vi "函数类型1测试.vi"() -> ()   [LabVIEW 2010]
uses:
  全局量/试验配置信息.vi
  全局量/全局_配置.vi
panel:
  in  "配置文件列表":u16(ring)
  in  "同步_1":i32
  in  "数组_反馈值":dbl[][](array[numeric])
  in  "第几个数据":i32
  in  "第几组数据":i32
  out "数组_AD幅值":sgl[](array[numeric])
  out "数组_DSP幅值":sgl[](array[numeric])
  in  "数组_设定值":dbl[][](array[numeric])
  in  "数组_选择":bool[](array[boolean])
  out "light_32":bool
  out "light_31":bool
  out "light_30":bool
  out "light_29":bool
  out "light_28":bool
  out "light_27":bool
  out "light_26":bool
  out "light_25":bool
  out "light_24":bool
  out "light_23":bool
  out "light_22":bool
  out "light_21":bool
  out "light_20":bool
  out "light_19":bool
  out "light_18":bool
  out "light_17":bool
  out "Analog_back":string[][](table) caption="表格"
  in  "A_32":bool
  in  "A_31":bool
  in  "A_30":bool
  in  "A_29":bool
  in  "A_28":bool
  in  "A_27":bool
  in  "A_26":bool
  in  "A_25":bool
  in  "A_24":bool
  in  "A_23":bool
  in  "A_22":bool
  in  "A_21":bool
  in  "A_20":bool
  in  "A_19":bool
  in  "A_18":bool
  in  "A_17":bool
  out "合格？":bool[][](array[boolean])
  out "测试结论":string
  out "light_16":bool
  out "light_15":bool
  out "light_14":bool
  out "light_13":bool
  out "light_12":bool
  out "light_11":bool
  out "light_10":bool
  out "light_9":bool
  out "light_8":bool
  out "light_7":bool
  out "light_6":bool
  out "light_5":bool
  out "light_4":bool
  out "light_3":bool
  out "light_2":bool
  out "light_1":bool
  out "退出？":bool
  in  "btn_反选":bool
  in  "btn_全选":bool
  in  "A_16":bool
  in  "A_15":bool
  in  "A_14":bool
  in  "A_13":bool
  in  "A_12":bool
  in  "A_11":bool
  in  "A_10":bool
  in  "A_9":bool
  in  "A_8":bool
  in  "A_7":bool
  in  "A_6":bool
  in  "A_5":bool
  in  "A_4":bool
  in  "A_3":bool
  in  "A_2":bool
  in  "A_1":bool
  in  "btn_取消":bool
  in  "btn_开始测试":bool
  in  "Analog_IN":string[][](table) caption="表格"
  out "Analog_WC":string[][](table) caption="表格"
  # "模拟量选择及输入值（V）"
  # "模拟量反馈值（V）"
  # "模拟量误差值（%）"
  # "加载配置文件："
  # "测试结论："
  # "从0开始"
  # "从1开始,第0列没有使用"
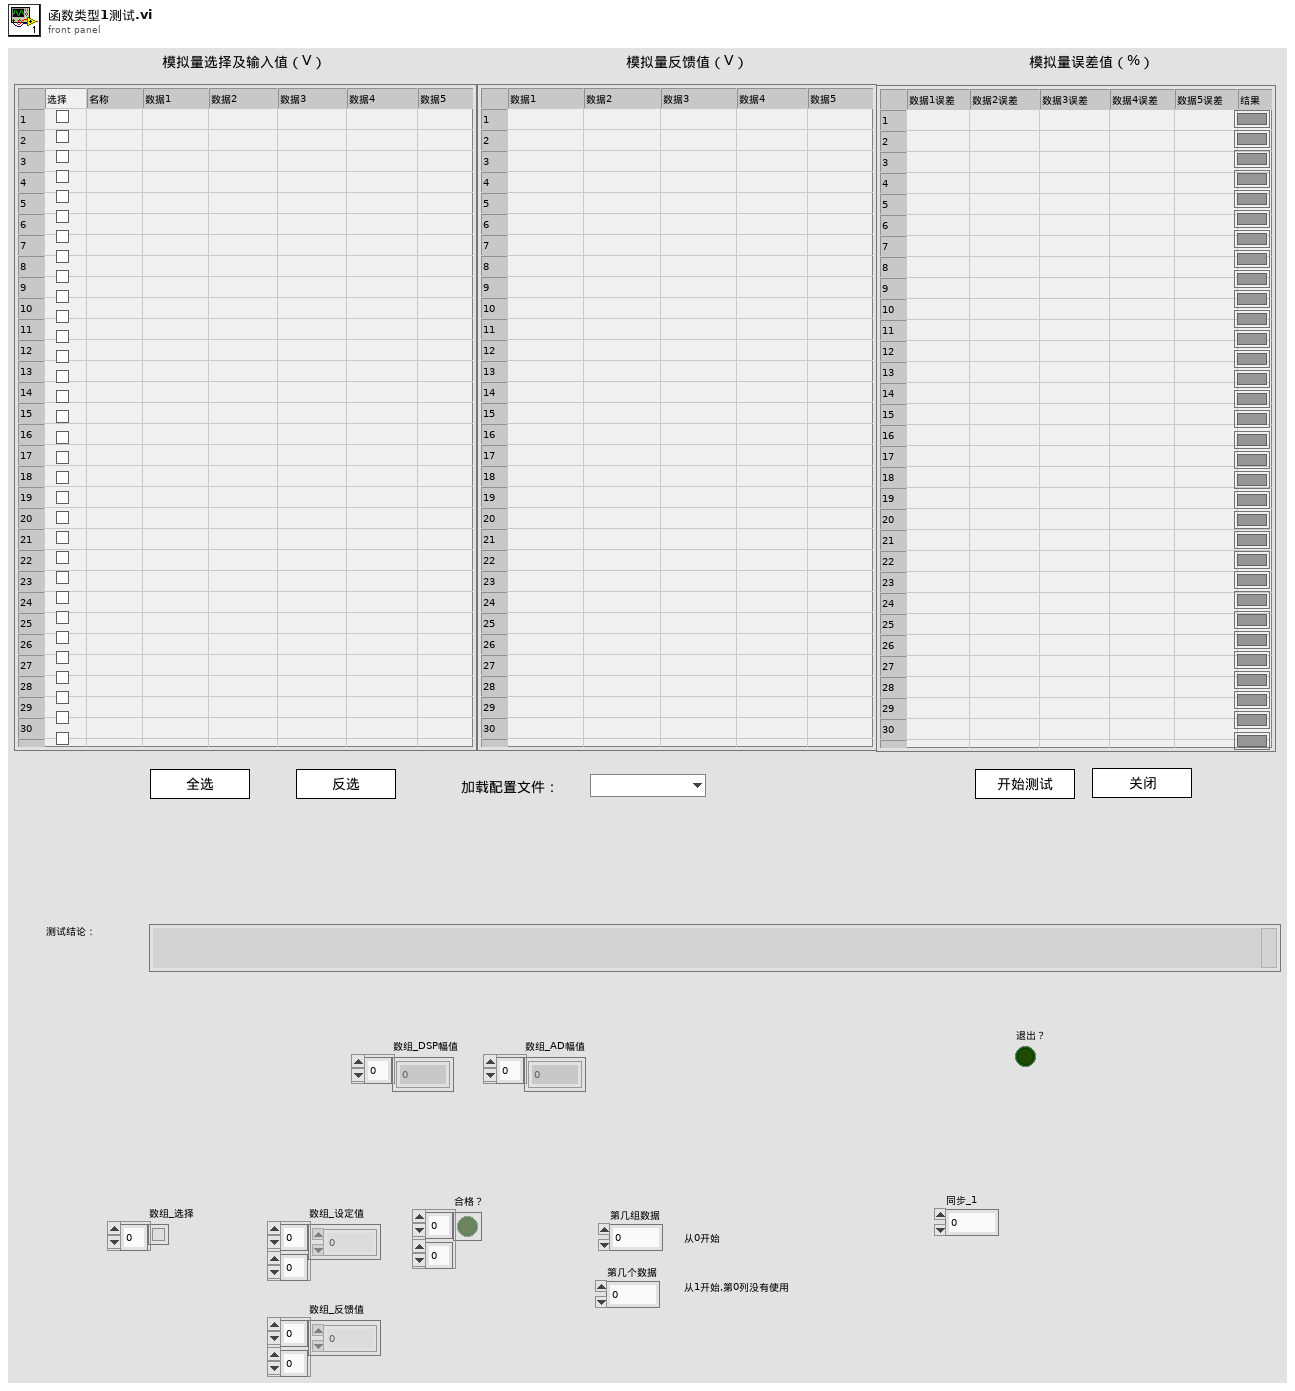
[diagram p1: front panel]
types:
  T1 = enum8{"Enabled", "Disabled", "Disabled and Grayed Out"}
  T2 = cluster{"数字量输入信号路数":u32, "数字量输出信号路数":u32, "DSP模拟量输入信号路数":u32, "DSP模拟量输入信号幅值":u32, "AD模拟量输入信号路数":u32, "AD模拟量输入信号幅值":u32, "RS232端口":u32, "RS232通信路数":u32, "RS232波特率":u32, "RS485端口":u32, "RS485通信路数":u32, "RS485波特率":u32, "CAN通信端口":string, "CAN波特率":u32, "以太网选择?":bool, "控制板IP":string, "以太网端口":u32}
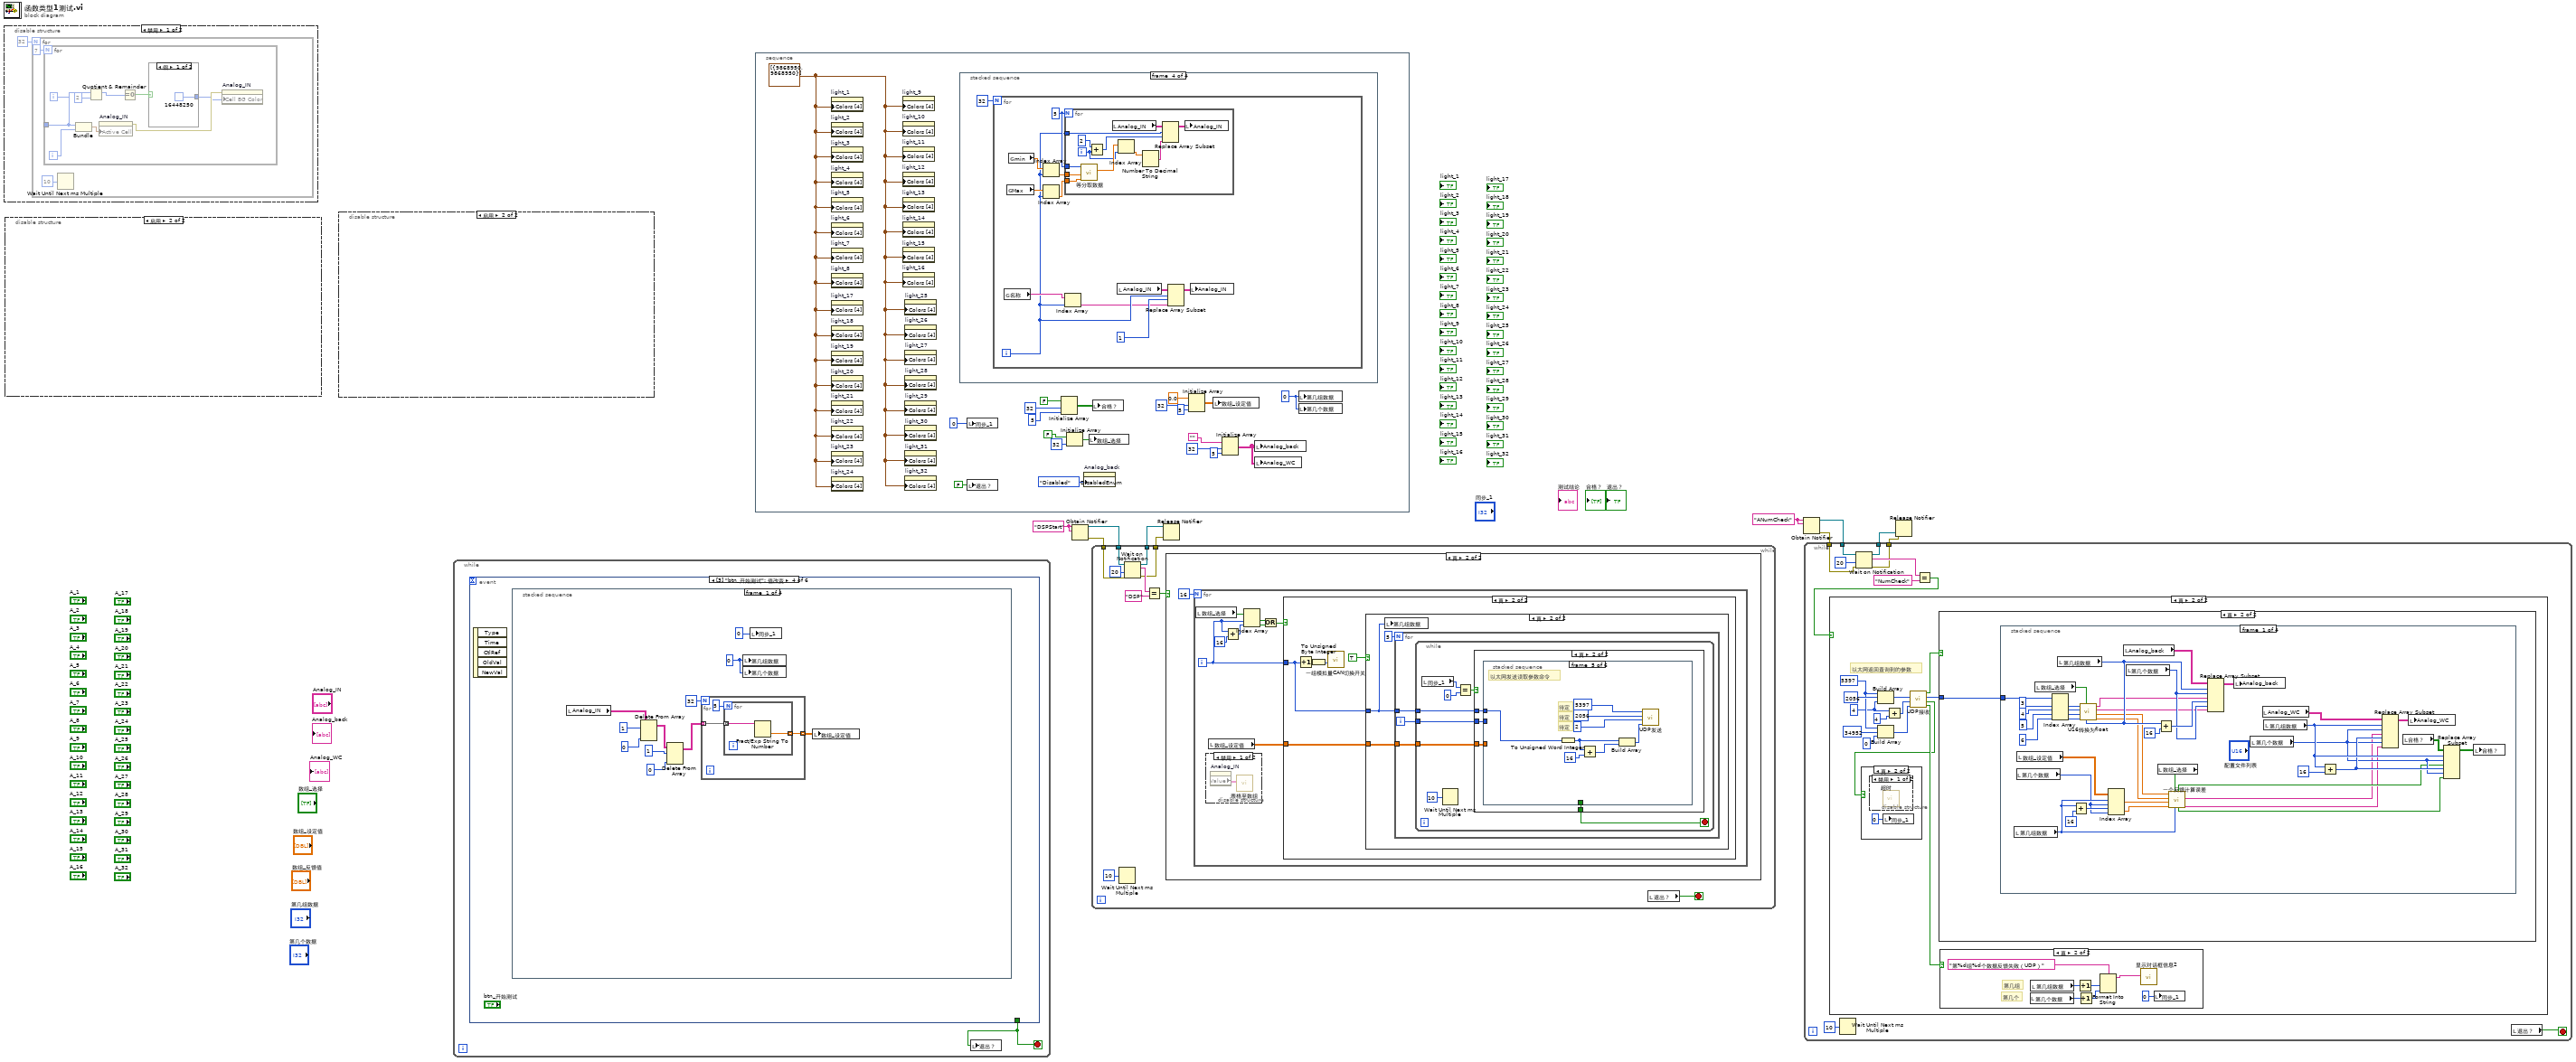
[diagram p0: block diagram]
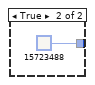
[diagram p2: hidden frame]
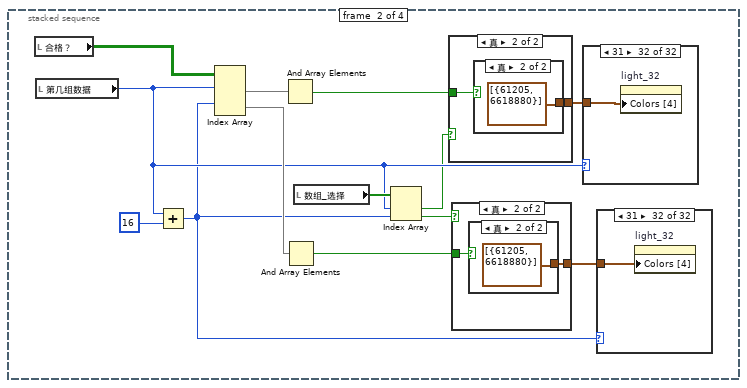
[diagram p9: hidden frame]
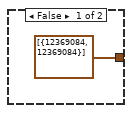
[diagram p10: hidden frame]
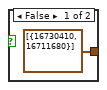
[diagram p11: hidden frame]
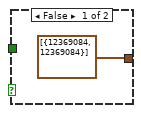
[diagram p12: hidden frame]
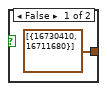
[diagram p13: hidden frame]
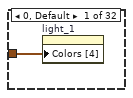
[diagram p14: hidden frame]
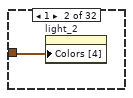
[diagram p15: hidden frame]
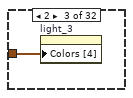
[diagram p16: hidden frame]
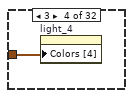
[diagram p17: hidden frame]
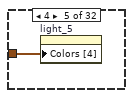
[diagram p18: hidden frame]
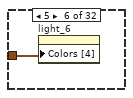
[diagram p19: hidden frame]
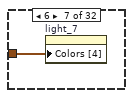
[diagram p20: hidden frame]
diagram:
  w5 = "ANumCheck" ("名称（未命名）")
  w8 = "DSPStart" ("名称（未命名）")
  n1 = disable-structure shown="禁用" {
    frame Disabled {
      n2 = for {
        N: 32 -> [_]
        i -> [w13]
        n3 = for {
          N: 7 -> [_]
          tunnel: w13 -> [w21]
          i -> [w15]
          n4 = Bundle(w21, w15) -> (w18:cluster{i32, i32})  [unwired: 1 in]
          n5 = Quotient & Remainder(x=w21, y=2) -> (x-y*floor(x/y)=w19:i32)  [unwired: 1 out]
          n6 = property on="Analog_IN" class="Tbl (严格)"("Active Cell"=w18) -> (error out=w17:errorcluster)  [unwired: 2 in, 1 out]
          n7 = Equal To 0?(x=w19) -> (x = 0?=w22:bool)
          n8 = case shown="假" w22 {
            tunnel: [u32 16448250 u32 15723488] -> w16
            frame False {
            }
            frame True {
            }
          }
          n9 = property on="Analog_IN" class="Tbl (严格)"(error in=w17, "Cell BG Color"=w16) -> ()  [unwired: 1 in, 2 out]
        }
        n10 = Wait Until Next ms Multiple(millisecond multiple=u32 10 ("毫秒倍数")) -> ()  [unwired: 1 out]
      }
    }
    frame Enabled {
    }
  }
  n11 = disable-structure shown="启用" {
    frame Disabled {
      n12 = for {
        N: 32 -> [_]
        i -> [w26]
        n13 = for {
          N: 7 -> [_]
          tunnel: w26 -> [w29]
          i -> [w30]
          n14 = Bundle(w29, w30) -> (w33:cluster{i32, i32})  [unwired: 1 in]
          n15 = property on="Analog_IN" class="Tbl (严格)"("Active Cell"=w33) -> (error out=w31:errorcluster)  [unwired: 2 in, 1 out]
          n16 = property on="Analog_IN" class="Tbl (严格)"(error in=w31, "Justify"=enum16{"Left", "Center", "Right"}."Left" ("活动单元格:单元格对齐")) -> ()  [unwired: 1 in, 2 out]
        }
        n17 = Wait Until Next ms Multiple(millisecond multiple=u32 10 ("毫秒倍数")) -> ()  [unwired: 1 out]
      }
    }
    frame Enabled {
    }
  }
  n18 = disable-structure shown="启用" {
    frame Disabled {
      n19 = for {
        N: 32 -> [_]
        i -> [w39]
        n20 = Wait Until Next ms Multiple(millisecond multiple=u32 10 ("毫秒倍数")) -> ()  [unwired: 1 out]
        n21 = Bundle(w39, 1) -> (w38:cluster{i32, i32})  [unwired: 1 in]
        n22 = property on="Analog_IN" class="Tbl (严格)"("Active Cell"=w38) -> (error out=w35:errorcluster)  [unwired: 2 in, 1 out]
        n23 = property on="Analog_IN" class="Tbl (严格)"(error in=w35, "DisabledEnum"=T1."Enabled" ("禁用")) -> ()  [unwired: 1 in, 2 out]
      }
    }
    frame Enabled {
    }
  }
  n24 = while {
    stop <- w41 stop-if-true
    n25 = event shown="[3] \"btn_开始测试\": 值改变" {
      selector: _ -> [_ _ _ _ _ _]
      dyn-events: _ -> [_ _ _ _ _ _]
      timeout: _ -> [_ _ _ _ _ _]
      tunnel: [_ TRUE TRUE _ _ _] -> w41
      event Timeout {
        n26 = event-data() -> ()  [unwired: 1 in, 2 out]
      }
      event Panel Close {
        n27 = event-data() -> ()  [unwired: 1 in, 3 out]
      }
      event "btn_取消": Value Change {
        n28 = event-data() -> ()  [unwired: 1 in, 5 out]
      }
      event "btn_开始测试": Value Change {
        n29 = event-data() -> ()  [unwired: 1 in, 5 out]
        n30 = stacked-sequence {
          frame #0 {
            w48 = 0 ("第几组数据")
            n31 = local read "Analog_IN"() -> (w54:string[][])
            n32 = Delete From Array(array=w54, length=1 ("长度"), index (col)=0 ("禁用的索引 (列)")) -> (array with subset deleted=w46:string[][])  [unwired: 1 in, 1 out]
            n33 = Delete From Array(array=w46, length=1 ("长度"), index (col)=0 ("禁用的索引 (列)")) -> (array with subset deleted=w44:string[][])  [unwired: 1 in, 1 out]
            n34 = for {
              N: 32 -> [_]
              tunnel: w44 -> [w57] mode=indexing
              tunnel: [w56] -> w53 mode=indexing
              n35 = for {
                N: 5 -> [_]
                tunnel: w57 -> [w59] mode=indexing
                tunnel: [w58] -> w56 mode=indexing
                n36 = Fract/Exp String To Number(string=w59) -> (number=w58:dbl)  [unwired: 3 in, 1 out]
              }
            }
            n37 = local write "第几组数据"(w48) -> ()
            n38 = local write "第几个数据"(w48) -> ()
            n39 = local write "同步_1"(0 ("同步_2")) -> ()
            n40 = local write "数组_设定值"(w53) -> ()
          }
          frame #1 {
            n41 = local read "Analog_back"() -> (w62:string[][])
            n42 = local read "Analog_WC"() -> (w61:string[][])
            n43 = for {
              tunnel: w61 -> [w98] mode=indexing
              i -> [w97]
              n44 = for {
                tunnel: w98 -> [_] mode=indexing
                tunnel: w97 -> [w102]
                i -> [w101]
                n45 = local read "Analog_WC"() -> (w103:string[][])
                n46 = Replace Array Subset(array=w103, new element="", index (row)=w102, index (col)=w101) -> (w99:string[][])
                n47 = local write "Analog_WC"(w99) -> ()
              }
            }
            n48 = for {
              tunnel: w62 -> [w105] mode=indexing
              i -> [w104]
              n49 = for {
                tunnel: w105 -> [_] mode=indexing
                tunnel: w104 -> [w109]
                i -> [w108]
                n50 = local read "Analog_back"() -> (w110:string[][])
                n51 = Replace Array Subset(array=w110, new element="", index (row)=w109, index (col)=w108) -> (w106:string[][])
                n52 = local write "Analog_back"(w106) -> ()
              }
            }
            n53 = for {
              N: 32 -> [_]
              i -> [w64]
              n54 = case shown="31" w64 {
                tunnel: cluster{u32, u32}[] [{9868950, 9868950}] -> [w65 w66 w67 w68 w69 w70 w71 w72 w73 w74 w75 w76 w77 w78 w79 w80 w81 w82 w83 w84 w85 w86 w87 w88 w89 w90 w91 w92 w93 w94 w95 w96]
                frame 0, Default {
                  n55 = property on="light_1" class="Bool (严格)"("Colors [4]"=w65) -> ()  [unwired: 2 in, 2 out]
                }
                frame 1 {
                  n56 = property on="light_2" class="Bool (严格)"("Colors [4]"=w66) -> ()  [unwired: 2 in, 2 out]
                }
                frame 2 {
                  n57 = property on="light_3" class="Bool (严格)"("Colors [4]"=w67) -> ()  [unwired: 2 in, 2 out]
                }
                frame 3 {
                  n58 = property on="light_4" class="Bool (严格)"("Colors [4]"=w68) -> ()  [unwired: 2 in, 2 out]
                }
                frame 4 {
                  n59 = property on="light_5" class="Bool (严格)"("Colors [4]"=w69) -> ()  [unwired: 2 in, 2 out]
                }
                frame 5 {
                  n60 = property on="light_6" class="Bool (严格)"("Colors [4]"=w70) -> ()  [unwired: 2 in, 2 out]
                }
                frame 6 {
                  n61 = property on="light_7" class="Bool (严格)"("Colors [4]"=w71) -> ()  [unwired: 2 in, 2 out]
                }
                frame 7 {
                  n62 = property on="light_8" class="Bool (严格)"("Colors [4]"=w72) -> ()  [unwired: 2 in, 2 out]
                }
                frame 8 {
                  n63 = property on="light_9" class="Bool (严格)"("Colors [4]"=w73) -> ()  [unwired: 2 in, 2 out]
                }
                frame 9 {
                  n64 = property on="light_10" class="Bool (严格)"("Colors [4]"=w74) -> ()  [unwired: 2 in, 2 out]
                }
                frame 10 {
                  n65 = property on="light_11" class="Bool (严格)"("Colors [4]"=w75) -> ()  [unwired: 2 in, 2 out]
                }
                frame 11 {
                  n66 = property on="light_12" class="Bool (严格)"("Colors [4]"=w76) -> ()  [unwired: 2 in, 2 out]
                }
                frame 12 {
                  n67 = property on="light_13" class="Bool (严格)"("Colors [4]"=w77) -> ()  [unwired: 2 in, 2 out]
                }
                frame 13 {
                  n68 = property on="light_14" class="Bool (严格)"("Colors [4]"=w78) -> ()  [unwired: 2 in, 2 out]
                }
                frame 14 {
                  n69 = property on="light_15" class="Bool (严格)"("Colors [4]"=w79) -> ()  [unwired: 2 in, 2 out]
                }
                frame 15 {
                  n70 = property on="light_16" class="Bool (严格)"("Colors [4]"=w80) -> ()  [unwired: 2 in, 2 out]
                }
                frame 16 {
                  n71 = property on="light_17" class="Bool (严格)"("Colors [4]"=w81) -> ()  [unwired: 2 in, 2 out]
                }
                frame 17 {
                  n72 = property on="light_18" class="Bool (严格)"("Colors [4]"=w82) -> ()  [unwired: 2 in, 2 out]
                }
                frame 18 {
                  n73 = property on="light_19" class="Bool (严格)"("Colors [4]"=w83) -> ()  [unwired: 2 in, 2 out]
                }
                frame 19 {
                  n74 = property on="light_20" class="Bool (严格)"("Colors [4]"=w84) -> ()  [unwired: 2 in, 2 out]
                }
                frame 20 {
                  n75 = property on="light_21" class="Bool (严格)"("Colors [4]"=w85) -> ()  [unwired: 2 in, 2 out]
                }
                frame 21 {
                  n76 = property on="light_22" class="Bool (严格)"("Colors [4]"=w86) -> ()  [unwired: 2 in, 2 out]
                }
                frame 22 {
                  n77 = property on="light_23" class="Bool (严格)"("Colors [4]"=w87) -> ()  [unwired: 2 in, 2 out]
                }
                frame 23 {
                  n78 = property on="light_24" class="Bool (严格)"("Colors [4]"=w88) -> ()  [unwired: 2 in, 2 out]
                }
                frame 24 {
                  n79 = property on="light_25" class="Bool (严格)"("Colors [4]"=w89) -> ()  [unwired: 2 in, 2 out]
                }
                frame 25 {
                  n80 = property on="light_26" class="Bool (严格)"("Colors [4]"=w90) -> ()  [unwired: 2 in, 2 out]
                }
                frame 26 {
                  n81 = property on="light_27" class="Bool (严格)"("Colors [4]"=w91) -> ()  [unwired: 2 in, 2 out]
                }
                frame 27 {
                  n82 = property on="light_28" class="Bool (严格)"("Colors [4]"=w92) -> ()  [unwired: 2 in, 2 out]
                }
                frame 28 {
                  n83 = property on="light_29" class="Bool (严格)"("Colors [4]"=w93) -> ()  [unwired: 2 in, 2 out]
                }
                frame 29 {
                  n84 = property on="light_30" class="Bool (严格)"("Colors [4]"=w94) -> ()  [unwired: 2 in, 2 out]
                }
                frame 30 {
                  n85 = property on="light_31" class="Bool (严格)"("Colors [4]"=w95) -> ()  [unwired: 2 in, 2 out]
                }
                frame 31 {
                  n86 = property on="light_32" class="Bool (严格)"("Colors [4]"=w96) -> ()  [unwired: 2 in, 2 out]
                }
              }
            }
          }
          frame #2 {
            n87 = for {
              N: 32 -> [_]
              i -> [w113]
              n88 = disable-structure shown="禁用" {
                frame Disabled {
                  n89 = Wait Until Next ms Multiple(millisecond multiple=u32 10 ("毫秒倍数")) -> ()  [unwired: 1 out]
                }
                frame Enabled {
                }
              }
              n90 = for {
                N: 6 -> [_]
                tunnel: w113 -> [w121]
                i -> [w118]
                n91 = Bundle(w121, w118) -> (w117:cluster{i32, i32})  [unwired: 1 in]
                n92 = Quotient & Remainder(x=w121, y=2) -> (x-y*floor(x/y)=w119:i32)  [unwired: 1 out]
                n93 = property on="Analog_WC" class="Tbl (严格)"("Active Cell"=w117) -> (error out=w116:errorcluster)  [unwired: 2 in, 1 out]
                n94 = Equal To 0?(x=w119) -> (x = 0?=w122:bool)
                n95 = case shown="假" w122 {
                  tunnel: [u32 16448250 u32 15723488] -> w115
                  frame False {
                  }
                  frame True {
                  }
                }
                n96 = property on="Analog_WC" class="Tbl (严格)"(error in=w116, "Cell BG Color"=w115) -> ()  [unwired: 1 in, 2 out]
              }
            }
          }
          frame #3 {
            n97 = local read "A_10"() -> (w153:bool)
            n98 = local read "A_11"() -> (w152:bool)
            n99 = local read "A_12"() -> (w151:bool)
            n100 = local read "A_13"() -> (w150:bool)
            n101 = local read "A_14"() -> (w149:bool)
            n102 = local read "A_15"() -> (w148:bool)
            n103 = local read "A_16"() -> (w147:bool)
            n104 = local read "A_17"() -> (w146:bool)
            n105 = local read "A_18"() -> (w145:bool)
            n106 = local read "A_19"() -> (w144:bool)
            n107 = local read "A_20"() -> (w143:bool)
            n108 = local read "A_21"() -> (w142:bool)
            n109 = local read "A_22"() -> (w141:bool)
            n110 = local read "A_23"() -> (w140:bool)
            n111 = local read "A_24"() -> (w139:bool)
            n112 = local read "A_25"() -> (w138:bool)
            n113 = local read "A_26"() -> (w137:bool)
            n114 = local read "A_27"() -> (w136:bool)
            n115 = local read "A_28"() -> (w135:bool)
            n116 = local read "A_29"() -> (w134:bool)
            n117 = local read "A_30"() -> (w133:bool)
            n118 = local read "A_31"() -> (w132:bool)
            n119 = local read "A_32"() -> (w131:bool)
            n120 = local read "A_1"() -> (w162:bool)
            n121 = local read "A_2"() -> (w161:bool)
            n122 = local read "A_3"() -> (w160:bool)
            n123 = local read "A_4"() -> (w159:bool)
            n124 = local read "A_5"() -> (w158:bool)
            n125 = local read "A_6"() -> (w157:bool)
            n126 = local read "A_7"() -> (w156:bool)
            n127 = local read "A_8"() -> (w155:bool)
            n128 = local read "A_9"() -> (w154:bool)
            n129 = Build Array(w162, w161, w160, w159, w158, w157, w156, w155, w154, w153, w152, w151, w150, w149, w148, w147, w146, w145, w144, w143, w142, w141, w140, w139, w138, w137, w136, w135, w134, w133, w132, w131) -> (w125:bool[])
            n130 = Or Array Elements(Boolean array=w125) -> (logical OR=w130:bool)
            n131 = case shown="真" w130 {
              frame False {
                n132 = call "显示对话框信息"() -> ()  [unwired: 10 in, 2 out]
              }
              frame True {
                w164 = "DSPStart" ("名称（未命名）")
                n133 = Obtain Notifier(name (unnamed)=w164, notification data type=w164) -> (notifier out=w163:refnum<notifier>)  [unwired: 2 in, 2 out]
                n134 = Send Notification(notification="DSP" ("通知"), notifier=w163) -> ()  [unwired: 1 in, 2 out]
              }
            }
            n135 = local write "数组_选择"(w125) -> ()
            n136 = Initialize Array(FALSE, 32 ("维数大小"), 5 ("维数大小")) -> (w126:bool[][])
            n137 = local write "合格？"(w126) -> ()
          }
        }
      }
      event "btn_全选": Value Change {
        w166 = TRUE ("单选_AD_1")
        n138 = event-data() -> ()  [unwired: 1 in, 5 out]
        n139 = local write "A_1"(w166) -> ()
        n140 = local write "A_2"(w166) -> ()
        n141 = local write "A_3"(w166) -> ()
        n142 = local write "A_4"(w166) -> ()
        n143 = local write "A_5"(w166) -> ()
        n144 = local write "A_6"(w166) -> ()
        n145 = local write "A_7"(w166) -> ()
        n146 = local write "A_8"(w166) -> ()
        n147 = local write "A_9"(w166) -> ()
        n148 = local write "A_10"(w166) -> ()
        n149 = local write "A_11"(w166) -> ()
        n150 = local write "A_12"(w166) -> ()
        n151 = local write "A_13"(w166) -> ()
        n152 = local write "A_14"(w166) -> ()
        n153 = local write "A_15"(w166) -> ()
        n154 = local write "A_16"(w166) -> ()
        n155 = local write "A_17"(w166) -> ()
        n156 = local write "A_18"(w166) -> ()
        n157 = local write "A_19"(w166) -> ()
        n158 = local write "A_20"(w166) -> ()
        n159 = local write "A_21"(w166) -> ()
        n160 = local write "A_22"(w166) -> ()
        n161 = local write "A_23"(w166) -> ()
        n162 = local write "A_24"(w166) -> ()
        n163 = local write "A_25"(w166) -> ()
        n164 = local write "A_26"(w166) -> ()
        n165 = local write "A_27"(w166) -> ()
        n166 = local write "A_28"(w166) -> ()
        n167 = local write "A_29"(w166) -> ()
        n168 = local write "A_30"(w166) -> ()
        n169 = local write "A_31"(w166) -> ()
        n170 = local write "A_32"(w166) -> ()
      }
      event "btn_反选": Value Change {
        n171 = event-data() -> ()  [unwired: 1 in, 5 out]
        n172 = local read "A_17"() -> (w198:bool)
        n173 = local read "A_18"() -> (w196:bool)
        n174 = local read "A_19"() -> (w194:bool)
        n175 = local read "A_20"() -> (w192:bool)
        n176 = local read "A_21"() -> (w190:bool)
        n177 = local read "A_22"() -> (w188:bool)
        n178 = local read "A_23"() -> (w186:bool)
        n179 = local read "A_24"() -> (w184:bool)
        n180 = local read "A_25"() -> (w182:bool)
        n181 = local read "A_26"() -> (w180:bool)
        n182 = local read "A_27"() -> (w178:bool)
        n183 = local read "A_28"() -> (w176:bool)
        n184 = local read "A_29"() -> (w174:bool)
        n185 = local read "A_30"() -> (w172:bool)
        n186 = local read "A_31"() -> (w170:bool)
        n187 = local read "A_32"() -> (w168:bool)
        n188 = local read "A_1"() -> (w230:bool)
        n189 = local read "A_2"() -> (w228:bool)
        n190 = local read "A_3"() -> (w227:bool)
        n191 = local read "A_4"() -> (w226:bool)
        n192 = local read "A_5"() -> (w225:bool)
        n193 = local read "A_6"() -> (w224:bool)
        n194 = local read "A_7"() -> (w223:bool)
        n195 = local read "A_8"() -> (w222:bool)
        n196 = local read "A_9"() -> (w221:bool)
        n197 = local read "A_10"() -> (w220:bool)
        n198 = local read "A_11"() -> (w219:bool)
        n199 = local read "A_12"() -> (w218:bool)
        n200 = local read "A_13"() -> (w217:bool)
        n201 = local read "A_14"() -> (w216:bool)
        n202 = local read "A_15"() -> (w215:bool)
        n203 = local read "A_16"() -> (w214:bool)
        n204 = Not(x=w230) -> (.not. x?=w229:bool)
        n205 = Not(x=w228) -> (.not. x?=w199:bool)
        n206 = Not(x=w227) -> (.not. x?=w200:bool)
        n207 = Not(x=w226) -> (.not. x?=w201:bool)
        n208 = Not(x=w225) -> (.not. x?=w202:bool)
        n209 = Not(x=w224) -> (.not. x?=w203:bool)
        n210 = Not(x=w223) -> (.not. x?=w204:bool)
        n211 = Not(x=w222) -> (.not. x?=w205:bool)
        n212 = Not(x=w221) -> (.not. x?=w206:bool)
        n213 = Not(x=w220) -> (.not. x?=w207:bool)
        n214 = Not(x=w219) -> (.not. x?=w208:bool)
        n215 = Not(x=w218) -> (.not. x?=w209:bool)
        n216 = Not(x=w217) -> (.not. x?=w210:bool)
        n217 = Not(x=w216) -> (.not. x?=w211:bool)
        n218 = Not(x=w215) -> (.not. x?=w212:bool)
        n219 = Not(x=w214) -> (.not. x?=w213:bool)
        n220 = Not(x=w198) -> (.not. x?=w197:bool)
        n221 = Not(x=w196) -> (.not. x?=w195:bool)
        n222 = Not(x=w194) -> (.not. x?=w193:bool)
        n223 = Not(x=w192) -> (.not. x?=w191:bool)
        n224 = Not(x=w190) -> (.not. x?=w189:bool)
        n225 = Not(x=w188) -> (.not. x?=w187:bool)
        n226 = Not(x=w186) -> (.not. x?=w185:bool)
        n227 = Not(x=w184) -> (.not. x?=w183:bool)
        n228 = Not(x=w182) -> (.not. x?=w181:bool)
        n229 = Not(x=w180) -> (.not. x?=w179:bool)
        n230 = Not(x=w178) -> (.not. x?=w177:bool)
        n231 = Not(x=w176) -> (.not. x?=w175:bool)
        n232 = Not(x=w174) -> (.not. x?=w173:bool)
        n233 = Not(x=w172) -> (.not. x?=w171:bool)
        n234 = Not(x=w170) -> (.not. x?=w169:bool)
        n235 = Not(x=w168) -> (.not. x?=w167:bool)
        n236 = local write "A_1"(w229) -> ()
        n237 = local write "A_2"(w199) -> ()
        n238 = local write "A_3"(w200) -> ()
        n239 = local write "A_4"(w201) -> ()
        n240 = local write "A_5"(w202) -> ()
        n241 = local write "A_6"(w203) -> ()
        n242 = local write "A_7"(w204) -> ()
        n243 = local write "A_8"(w205) -> ()
        n244 = local write "A_9"(w206) -> ()
        n245 = local write "A_10"(w207) -> ()
        n246 = local write "A_11"(w208) -> ()
        n247 = local write "A_12"(w209) -> ()
        n248 = local write "A_13"(w210) -> ()
        n249 = local write "A_14"(w211) -> ()
        n250 = local write "A_15"(w212) -> ()
        n251 = local write "A_16"(w213) -> ()
        n252 = local write "A_17"(w197) -> ()
        n253 = local write "A_18"(w195) -> ()
        n254 = local write "A_19"(w193) -> ()
        n255 = local write "A_20"(w191) -> ()
        n256 = local write "A_21"(w189) -> ()
        n257 = local write "A_22"(w187) -> ()
        n258 = local write "A_23"(w185) -> ()
        n259 = local write "A_24"(w183) -> ()
        n260 = local write "A_25"(w181) -> ()
        n261 = local write "A_26"(w179) -> ()
        n262 = local write "A_27"(w177) -> ()
        n263 = local write "A_28"(w175) -> ()
        n264 = local write "A_29"(w173) -> ()
        n265 = local write "A_30"(w171) -> ()
        n266 = local write "A_31"(w169) -> ()
        n267 = local write "A_32"(w167) -> ()
      }
    }
    n268 = local write "退出？"(w41) -> ()
  }
  n269 = stacked-sequence {
    frame #0 {
      w231 = 0 ("第几组数据")
      w246 = cluster{u32, u32}[] [{9868950, 9868950}]
      n270 = property on="light_1" class="Bool (严格)"("Colors [4]"=w246) -> ()  [unwired: 2 in, 2 out]
      n271 = property on="light_2" class="Bool (严格)"("Colors [4]"=w246) -> ()  [unwired: 2 in, 2 out]
      n272 = property on="light_3" class="Bool (严格)"("Colors [4]"=w246) -> ()  [unwired: 2 in, 2 out]
      n273 = property on="light_4" class="Bool (严格)"("Colors [4]"=w246) -> ()  [unwired: 2 in, 2 out]
      n274 = property on="light_5" class="Bool (严格)"("Colors [4]"=w246) -> ()  [unwired: 2 in, 2 out]
      n275 = property on="light_6" class="Bool (严格)"("Colors [4]"=w246) -> ()  [unwired: 2 in, 2 out]
      n276 = property on="light_7" class="Bool (严格)"("Colors [4]"=w246) -> ()  [unwired: 2 in, 2 out]
      n277 = property on="light_8" class="Bool (严格)"("Colors [4]"=w246) -> ()  [unwired: 2 in, 2 out]
      n278 = property on="light_17" class="Bool (严格)"("Colors [4]"=w246) -> ()  [unwired: 2 in, 2 out]
      n279 = property on="light_18" class="Bool (严格)"("Colors [4]"=w246) -> ()  [unwired: 2 in, 2 out]
      n280 = property on="light_19" class="Bool (严格)"("Colors [4]"=w246) -> ()  [unwired: 2 in, 2 out]
      n281 = property on="light_20" class="Bool (严格)"("Colors [4]"=w246) -> ()  [unwired: 2 in, 2 out]
      n282 = property on="light_21" class="Bool (严格)"("Colors [4]"=w246) -> ()  [unwired: 2 in, 2 out]
      n283 = property on="light_22" class="Bool (严格)"("Colors [4]"=w246) -> ()  [unwired: 2 in, 2 out]
      n284 = property on="light_23" class="Bool (严格)"("Colors [4]"=w246) -> ()  [unwired: 2 in, 2 out]
      n285 = property on="light_24" class="Bool (严格)"("Colors [4]"=w246) -> ()  [unwired: 2 in, 2 out]
      n286 = property on="light_9" class="Bool (严格)"("Colors [4]"=w246) -> ()  [unwired: 2 in, 2 out]
      n287 = property on="light_10" class="Bool (严格)"("Colors [4]"=w246) -> ()  [unwired: 2 in, 2 out]
      n288 = property on="light_11" class="Bool (严格)"("Colors [4]"=w246) -> ()  [unwired: 2 in, 2 out]
      n289 = property on="light_12" class="Bool (严格)"("Colors [4]"=w246) -> ()  [unwired: 2 in, 2 out]
      n290 = property on="light_13" class="Bool (严格)"("Colors [4]"=w246) -> ()  [unwired: 2 in, 2 out]
      n291 = property on="light_14" class="Bool (严格)"("Colors [4]"=w246) -> ()  [unwired: 2 in, 2 out]
      n292 = property on="light_15" class="Bool (严格)"("Colors [4]"=w246) -> ()  [unwired: 2 in, 2 out]
      n293 = property on="light_16" class="Bool (严格)"("Colors [4]"=w246) -> ()  [unwired: 2 in, 2 out]
      n294 = property on="light_25" class="Bool (严格)"("Colors [4]"=w246) -> ()  [unwired: 2 in, 2 out]
      n295 = property on="light_26" class="Bool (严格)"("Colors [4]"=w246) -> ()  [unwired: 2 in, 2 out]
      n296 = property on="light_27" class="Bool (严格)"("Colors [4]"=w246) -> ()  [unwired: 2 in, 2 out]
      n297 = property on="light_28" class="Bool (严格)"("Colors [4]"=w246) -> ()  [unwired: 2 in, 2 out]
      n298 = property on="light_29" class="Bool (严格)"("Colors [4]"=w246) -> ()  [unwired: 2 in, 2 out]
      n299 = property on="light_30" class="Bool (严格)"("Colors [4]"=w246) -> ()  [unwired: 2 in, 2 out]
      n300 = property on="light_31" class="Bool (严格)"("Colors [4]"=w246) -> ()  [unwired: 2 in, 2 out]
      n301 = property on="light_32" class="Bool (严格)"("Colors [4]"=w246) -> ()  [unwired: 2 in, 2 out]
      n302 = stacked-sequence {
        frame #0 {
          n303 = Initialize Array("", 32 ("维数大小"), 7 ("维数大小")) -> (w260:string[][])
          n304 = Initialize Array(-15.0 ("元素"), 32 ("维数大小")) -> (w254:dbl[])
          n305 = Initialize Array(15.0 ("元素"), 32 ("维数大小")) -> (w259:dbl[])
          n306 = Initialize Array("测试", 32 ("维数大小")) -> (w252:string[])
          n307 = local write "Analog_IN"(w260) -> ()
          n308 = global write "试验配置信息.vi" "min"(w254) -> ()
          n309 = global write "试验配置信息.vi" "Max"(w259) -> ()
          n310 = global write "试验配置信息.vi" "名称"(w252) -> ()
        }
        frame #1 {
          n311 = disable-structure shown="启用" {
            frame Disabled {
              n312 = global read "全局_配置.vi" "BoardConfig"() -> (w268:T2)
              n313 = Unbundle By Name(w268) -> ("DSP模拟量输入信号幅值"=w267:u32, "AD模拟量输入信号幅值"=w266:u32)
              n314 = case shown="1" w266 {
                tunnel: [sgl 3.0 sgl 5.0 sgl 12.0] -> w264
                frame 0, Default {
                }
                frame 1 {
                }
                frame 2 {
                }
              }
              n315 = case shown="2" w267 {
                tunnel: [sgl 3.0 sgl 5.0 sgl 12.0] -> w265
                frame 0, Default {
                }
                frame 1 {
                }
                frame 2 {
                }
              }
              n316 = for {
                N: 5 -> [_]
                tunnel: w265 -> [w290]
                tunnel: w264 -> [w281]
                tunnel: [w279] -> w270 mode=indexing
                tunnel: [w278] -> w269 mode=indexing
                i -> [w293]
                n317 = Multiply(x=sgl 2.0, y=w290) -> (x*y=w288:sgl)
                n318 = Multiply(x=sgl 2.0, y=w281) -> (x*y=w285:sgl)
                n319 = case shown="4" w293 {
                  tunnel: [sgl 0.05 sgl 0.5 sgl 0.75 sgl 0.95 sgl 0.25] -> w280
                  frame 0, Default {
                  }
                  frame 2 {
                  }
                  frame 3 {
                  }
                  frame 4 {
                  }
                  frame 1 {
                  }
                }
                n320 = Multiply(x=w290, y=sgl -1.0) -> (x*y=w291:sgl)
                n321 = Multiply(x=w281, y=sgl -1.0) -> (x*y=w283:sgl)
                n322 = Multiply(x=w280, y=w288) -> (x*y=w287:sgl)
                n323 = Multiply(x=w280, y=w285) -> (x*y=w286:sgl)
                n324 = Add(x=w287, y=w291) -> (x+y=w279:sgl)
                n325 = Add(x=w286, y=w283) -> (x+y=w278:sgl)
              }
              "数组_DSP幅值" <- w270
              "数组_AD幅值" <- w269
            }
            frame Enabled {
              n326 = Initialize Array(sgl 2.0, 5 ("维数大小")) -> (w301:sgl[])
              n327 = local write "数组_DSP幅值"(w301) -> ()
              n328 = local write "数组_AD幅值"(w301) -> ()
            }
          }
        }
        frame #2 {
          n329 = disable-structure shown="禁用" {
            frame Disabled {
              n330 = stacked-sequence {
                frame #0 {
                  n331 = for {
                    N: 16 -> [_]
                    i -> [w303]
                    n332 = local read "数组_DSP幅值"() -> (w304:sgl[])
                    n333 = for {
                      N: 5 -> [_]
                      tunnel: w304 -> [w312] mode=indexing
                      tunnel: w303 -> [w311]
                      i -> [w308]
                      w306 = i16 2 ("精度(6)")
                      n334 = local read "Analog_IN"() -> (w314:string[][])
                      n335 = Number To Fractional String(number=w312, precision (6)=w306) -> (F-format string=w310:string)  [unwired: 2 in]
                      n336 = Add(x=w308, y=w306) -> (x+y=w307:i32)
                      n337 = Replace Array Subset(array=w314, new element=w310, index (row)=w311, index (col)=w307) -> (w313:string[][])
                      n338 = local write "Analog_IN"(w313) -> ()
                      n339 = Wait Until Next ms Multiple(millisecond multiple=u32 2 ("毫秒倍数")) -> ()  [unwired: 1 out]
                    }
                  }
                }
                frame #1 {
                  n340 = for {
                    N: 16 -> [_]
                    i -> [w317]
                    n341 = local read "数组_AD幅值"() -> (w316:sgl[])
                    n342 = for {
                      N: 5 -> [_]
                      tunnel: w316 -> [w327] mode=indexing
                      tunnel: w317 -> [w324]
                      i -> [w321]
                      w320 = i16 2 ("精度(6)")
                      n343 = Add(x=w324, y=16) -> (x+y=w322:i32)
                      n344 = local read "Analog_IN"() -> (w329:string[][])
                      n345 = Add(x=w321, y=w320) -> (x+y=w319:i32)
                      n346 = Number To Fractional String(number=w327, precision (6)=w320) -> (F-format string=w326:string)  [unwired: 2 in]
                      n347 = Replace Array Subset(array=w329, new element=w326, index (row)=w322, index (col)=w319) -> (w328:string[][])
                      n348 = local write "Analog_IN"(w328) -> ()
                      n349 = Wait Until Next ms Multiple(millisecond multiple=u32 2 ("毫秒倍数")) -> ()  [unwired: 1 out]
                    }
                  }
                }
              }
            }
            frame Enabled {
            }
          }
        }
        frame #3 {
          n350 = for {
            N: 32 -> [_]
            i -> [w333]
            w337 = 5 ("num")
            n351 = global read "试验配置信息.vi" "名称"() -> (w336:string[])
            n352 = global read "试验配置信息.vi" "Max"() -> (w340:dbl[])
            n353 = global read "试验配置信息.vi" "min"() -> (w341:dbl[])
            n354 = Index Array(array=w341, index=w333) -> (element=w339:dbl)
            n355 = Index Array(array=w340, index=w333) -> (element=w338:dbl)
            n356 = for {
              N: w337 -> [_]
              tunnel: w333 -> [w351]
              tunnel: w339 -> [w348]
              tunnel: w338 -> [w347]
              tunnel: w337 -> [w346]
              i -> [w342]
              n357 = call "等分取数据.vi"("Max"=w347, "MIN"=w348, "num"=w346) -> ("数据点"=w345:dbl[])  [unwired: 5 in]
              n358 = Add(x=2, y=w342) -> (x+y=w349:i32)
              n359 = local read "Analog_IN"() -> (w353:string[][])
              n360 = Index Array(array=w345, index=w342) -> (element=w344:dbl)
              n361 = Number To Decimal String(number=w344) -> (decimal integer string=w343:string)  [unwired: 1 in]
              n362 = Replace Array Subset(array=w353, new element=w343, index (row)=w351, index (col)=w349) -> (w352:string[][])
              n363 = local write "Analog_IN"(w352) -> ()
            }
            n364 = Index Array(array=w336, index=w333) -> (element=w331:string)
            n365 = local read "Analog_IN"() -> (w334:string[][])
            n366 = Replace Array Subset(array=w334, new element=w331, index (row)=w333, index (col)=1) -> (w335:string[][])
            n367 = local write "Analog_IN"(w335) -> ()
          }
        }
      }
      n368 = local write "同步_1"(0 ("同步_2")) -> ()
      n369 = local write "退出？"(FALSE ("退出？")) -> ()
      n370 = Initialize Array(FALSE, 32 ("维数大小"), 5 ("维数大小")) -> (w247:bool[][])
      n371 = Initialize Array(FALSE, 32 ("维数大小")) -> (w235:bool[])
      n372 = property on="Analog_back" class="Tbl (严格)"("DisabledEnum"=T1."Disabled" ("禁用")) -> ()  [unwired: 2 in, 2 out]
      n373 = local write "数组_选择"(w235) -> ()
      n374 = local write "合格？"(w247) -> ()
      n375 = Initialize Array(0.0, 32 ("维数大小"), 5 ("维数大小")) -> (w238:dbl[][])
      n376 = local write "数组_设定值"(w238) -> ()
      n377 = Initialize Array("", 32 ("维数大小"), 5 ("维数大小")) -> (w242:string[][])
      n378 = local write "Analog_back"(w242) -> ()
      n379 = local write "Analog_WC"(w242) -> ()
      n380 = local write "第几组数据"(w231) -> ()
      n381 = local write "第几个数据"(w231) -> ()
    }
  }
  n382 = Obtain Notifier(name (unnamed)=w8, notification data type=w8) -> (notifier out=w10:refnum<notifier>, error out=w9:errorcluster)  [unwired: 2 in, 1 out]
  n383 = while {
    tunnel: w10 -> [w357]
    tunnel: w9 -> [w356]
    tunnel: [w355] -> w7
    tunnel: [w354] -> w6
    stop <- w359 stop-if-true
    n384 = Wait Until Next ms Multiple(millisecond multiple=u32 10 ("毫秒倍数")) -> ()  [unwired: 1 out]
    n385 = Wait on Notification(notifier=w357, timeout in ms (-1)=20 ("超时毫秒(-1)"), error in (no error)=w356) -> (notifier out=w355:refnum<notifier>, notification=w363:string, error out=w354:errorcluster)  [unwired: 1 in, 1 out]
    n386 = Equal?(x=w363, y="DSP" ("通知")) -> (x = y?=w360:bool)
    n387 = case shown="真" w360 {
      frame False {
      }
      frame True {
        n388 = for {
          N: 16 -> [_]
          i -> [w368]
          n389 = local read "数组_选择"() -> (w371:bool[])
          n390 = disable-structure shown="禁用" {
            frame Disabled {
              n391 = property on="Analog_IN" class="Tbl (严格)"() -> ("Value"=w373:string[][])  [unwired: 2 in, 2 out]
              n392 = call "表格至数组.vi"("表格控件"=w373) -> ()  [unwired: 10 in, 1 out]
            }
            frame Enabled {
            }
          }
          n393 = local read "数组_设定值"() -> (w372:dbl[][])
          n394 = Add(x=w368, y=16) -> (x+y=w369:i32)
          n395 = Index Array(array=w371, index #1=w368, index #2=w369) -> (element #1=w366:bool, element #2=w365:bool)
          n396 = Or(x=w366, y=w365) -> (x .or. y?=w370:bool)
          n397 = case shown="真" w370 {
            tunnel: w368 -> [_ w374]
            tunnel: w372 -> [_ w376]
            frame False {
            }
            frame True {
              n398 = Increment(x=w374) -> (x+1=w377:i32)
              n399 = To Unsigned Byte Integer(number=w377) -> (unsigned 8bit integer=w378:u8)
              n400 = call "一组模拟量CAN切换开关.vi"("第几组数据"=w378) -> ()  [unwired: 10 in, 1 out]
              n401 = case shown="真" TRUE {
                tunnel: w374 -> [_ w379]
                tunnel: w376 -> [_ w380]
                frame False {
                }
                frame True {
                  n402 = local write "第几组数据"(w379) -> ()
                  n403 = for {
                    N: 5 -> [_]
                    tunnel: w379 -> [w384]
                    tunnel: w380 -> [w383]
                    i -> [w382]
                    n404 = while {
                      tunnel: w384 -> [w392]
                      tunnel: w383 -> [w391]
                      tunnel: w382 -> [w390]
                      stop <- w387 stop-if-true
                      n405 = local read "同步_1"() -> (w388:i32)
                      n406 = Wait Until Next ms Multiple(millisecond multiple=u32 10 ("毫秒倍数")) -> ()  [unwired: 1 out]
                      n407 = Equal?(x=w388, y=0) -> (x = y?=w389:bool)
                      n408 = case shown="真" w389 {
                        tunnel: w392 -> [_ w397]
                        tunnel: w391 -> [_ w396]
                        tunnel: w390 -> [_ w395]
                        tunnel: [FALSE w394] -> w387
                        frame False {
                        }
                        frame True {
                          n409 = stacked-sequence {
                            tunnel: w397 -> [_ w403 _ _ w421 _]
                            tunnel: w396 -> [_ w406 _ _ _ _]
                            tunnel: w395 -> [_ w399 _ _ _ _]
                            tunnel: [_ _ _ _ _ w422] -> w394
                            frame #0 {
                              n410 = Wait (ms)(milliseconds to wait=u32 100) -> ()  [unwired: 1 out]
                            }
                            frame #1 {
                              # "PCI板卡下发模拟量数据"
                              n411 = To Long Integer(number=w403) -> (32bit integer=w402:i32)
                              n412 = local write "第几个数据"(w399) -> ()
                              n413 = Add(x=w402, y=16) -> (x+y=w404:i32)
                              n414 = Index Array(array=w406, index (row) #1=w402, index (col) #1=w399, index (row) #2=w404, index (col) #2=w399) -> (element #1=w401:dbl, element #2=w400:dbl)
                              n415 = Build Array(w401, w400) -> (w407:dbl[])
                              n416 = call "Convert to Dynamic Data"("Array"=w407) -> ("Dynamic Data Type"=w408:dynamicdata)  [unwired: 3 out]
                              n417 = call "DAQNavi Assistant"("data in(DDT)"=w408) -> ()  [unwired: 2 in, 17 out]
                            }
                            frame #2 {
                              w411 = "ANumCheck" ("名称（未命名）")
                              n418 = Obtain Notifier(name (unnamed)=w411, notification data type=w411) -> (notifier out=w410:refnum<notifier>)  [unwired: 2 in, 2 out]
                              n419 = local write "同步_1"(1 ("同步_1")) -> ()
                              n420 = Send Notification(notification="NumCheck" ("通知"), notifier=w410) -> ()  [unwired: 1 in, 2 out]
                            }
                            frame #3 {
                              n421 = Wait (ms)(milliseconds to wait=u32 150) -> ()  [unwired: 1 out]
                            }
                            frame #4 {
                              # "待定"
                              # "待定"
                              # "待定"
                              # "以太网发送读取参数命令"
                              n422 = To Unsigned Word Integer(number=w421) -> (unsigned 16bit integer=w417:u16)
                              n423 = Add(x=w417, y=u16 16) -> (x+y=w418:u16)
                              n424 = Build Array(w417, w418) -> (w420:u16[])
                              n425 = call "UDP发送.vi"("发送数据"=w420, "数据区字长"=u16 2, "报文类型"=u16 2056, "发送方标识"=u16 5397) -> ()  [unwired: 6 in, 1 out]
                            }
                            frame #5 {
                              n426 = local read "同步_1"() -> (w424:i32)
                              n427 = Equal?(x=w424, y=1) -> (x = y?=w422:bool)
                            }
                          }
                        }
                      }
                    }
                  }
                }
              }
            }
          }
        }
      }
    }
    n428 = local read "退出？"() -> (w359:bool)
  }
  n429 = Release Notifier(notifier=w7, error in (no error)=w6) -> ()  [unwired: 1 in, 3 out]
  n430 = Obtain Notifier(name (unnamed)=w5, notification data type=w5) -> (notifier out=w4:refnum<notifier>, error out=w3:errorcluster)  [unwired: 2 in, 1 out]
  n431 = while {
    tunnel: w4 -> [w429]
    tunnel: w3 -> [w428]
    tunnel: [w427] -> w2
    tunnel: [w426] -> w1
    stop <- w425 stop-if-true
    n432 = Wait Until Next ms Multiple(millisecond multiple=u32 10 ("毫秒倍数")) -> ()  [unwired: 1 out]
    n433 = Wait on Notification(notifier=w429, timeout in ms (-1)=20 ("超时毫秒(-1)"), error in (no error)=w428) -> (notifier out=w427:refnum<notifier>, notification=w432:string, error out=w426:errorcluster)  [unwired: 1 in, 1 out]
    n434 = Equal?(x=w432, y="NumCheck" ("通知")) -> (x = y?=w430:bool)
    n435 = case shown="真" w430 {
      frame False {
      }
      frame True {
        w437 = u16 4
        w446 = u16 5397
        # "以太网返回查询到的参数"
        n436 = Build Array(w446, u16 2056, w437) -> (w443:u16[])
        n437 = Build Array(w446, u16 34952, u16 0 ("元素")) -> (w442:u16[])
        n438 = Add(x=w437, y=u16 4) -> (x+y=w435:u16)
        n439 = call "UDP接收.vi"("匹配帧信息_异常"=w442, "长度"=w435, "匹配帧信息_正常"=w443) -> ("异常_找到?"=w439:bool, "接收超时?"=w438:bool, "接收的一帧数据"=w440:u16[], "正常_找到?"=w441:bool)  [unwired: 5 in]
        n440 = case shown="真" w438 {
          frame False {
          }
          frame True {
            n441 = disable-structure shown="禁用" {
              frame Disabled {
                n442 = call "超时"() -> ()  [unwired: 10 in, 2 out]
              }
              frame Enabled {
              }
            }
            n443 = local write "同步_1"(0 ("同步_1")) -> ()
          }
        }
        n444 = case shown="真" w441 {
          tunnel: w440 -> [_ w456]
          frame False {
          }
          frame True {
            n445 = stacked-sequence {
              tunnel: w456 -> [w496 _ _ _]
              frame #0 {
                n446 = local read "第几组数据"() -> (w464:i32)
                n447 = local read "第几个数据"() -> (w459:i32)
                n448 = local read "数组_设定值"() -> (w490:dbl[][])
                n449 = local read "数组_选择"() -> (w468:bool[])
                n450 = Index Array(array=w496, index #1=3 ("索引"), index #2=4 ("索引"), index #3=5 ("索引"), index #4=6 ("索引")) -> (element #1=w475:u16, element #2=w474:u16, element #3=w473:u16, element #4=w472:u16)
                n451 = local read "第几组数据"() -> (w471:i32)
                n452 = Add(x=w464, y=16) -> (x+y=w477:i32)
                n453 = call "U16转换为float.vi"("第几组数据"=w471, "选择?"=w468, "低16位_2"=w472, "高16位_2"=w473, "低16位_1"=w474, "高16位_1"=w475) -> ("反馈值2"=w466:dbl, "反馈值1"=w457:dbl, "反馈值字符_2"=w469:string, "反馈值字符_1"=w470:string)  [unwired: 2 in]
                n454 = Index Array(array=w490, index (row) #1=w464, index (col) #1=w459, index (row) #2=w477, index (col) #2=w459) -> (element #1=w458:dbl, element #2=w465:dbl)
                n455 = local read "Analog_back"() -> (w482:string[][])
                n456 = local read "第几个数据"() -> (w476:i32)
                n457 = local read "数组_选择"() -> (w467:bool[])
                n458 = Add(x=w471, y=16) -> (x+y=w480:i32)
                n459 = call "一个反馈计算误差.vi"("第几组"=w464, "选择?"=w467, "设定值_2"=w465, "设定值_1"=w458, "反馈值_2"=w466, "反馈值_1"=w457) -> ("字符串_误差_2"=w461:string, "字符串_误差_1"=w462:string, "合格_2?"=w460:bool, "合格_1?"=w463:bool)  [unwired: 2 out]
                n460 = Replace Array Subset(array=w482, new element #1=w470, index (row) #1=w471, index (col) #1=w476, new element #2=w469, index (row) #2=w480, index (col) #2=w476) -> (w481:string[][])
                n461 = local write "Analog_back"(w481) -> ()
                n462 = local read "第几个数据"() -> (w478:i32)
                n463 = local read "Analog_WC"() -> (w487:string[][])
                n464 = local read "第几组数据"() -> (w485:i32)
                n465 = Add(x=w485, y=16) -> (x+y=w479:i32)
                n466 = Replace Array Subset(array=w487, new element #1=w462, index (row) #1=w485, index (col) #1=w478, new element #2=w461, index (row) #2=w479, index (col) #2=w478) -> (w486:string[][])
                n467 = local read "合格？"() -> (w483:bool[][])
                n468 = local write "Analog_WC"(w486) -> ()
                n469 = Replace Array Subset(array=w483, new element #1=w463, index (row) #1=w485, index (col) #1=w478, new element #2=w460, index (row) #2=w479, index (col) #2=w478) -> (w484:bool[][])
                n470 = local write "合格？"(w484) -> ()
              }
              frame #1 {
                n471 = local read "合格？"() -> (w506:bool[][])
                n472 = local read "第几组数据"() -> (w500:i32)
                n473 = Add(x=w500, y=16) -> (x+y=w499:i32)
                n474 = Index Array(array=w506, index (row) #1=w500, index (row) #2=w499) -> (element #1=w509:bool[], element #2=w503:bool[])  [unwired: 2 in]
                n475 = And Array Elements(Boolean array=w509) -> (logical AND=w504:bool)
                n476 = And Array Elements(Boolean array=w503) -> (logical AND=w502:bool)
                n477 = local read "数组_选择"() -> (w501:bool[])
                n478 = Index Array(array=w501, index #1=w500, index #2=w499) -> (element #1=w498:bool, element #2=w497:bool)
                n479 = case shown="真" w498 {
                  tunnel: [cluster{u32, u32}[] [{12369084, 12369084}] w517] -> w508
                  tunnel: w504 -> [_ w516]
                  frame False {
                  }
                  frame True {
                    n480 = case shown="真" w516 {
                      tunnel: [cluster{u32, u32}[] [{16730410, 16711680}] cluster{u32, u32}[] [{61205, 6618880}]] -> w517
                      frame False {
                      }
                      frame True {
                      }
                    }
                  }
                }
                n481 = case shown="真" w497 {
                  tunnel: [cluster{u32, u32}[] [{12369084, 12369084}] w512] -> w505
                  tunnel: w502 -> [_ w511]
                  frame False {
                  }
                  frame True {
                    n482 = case shown="真" w511 {
                      tunnel: [cluster{u32, u32}[] [{16730410, 16711680}] cluster{u32, u32}[] [{61205, 6618880}]] -> w512
                      frame False {
                      }
                      frame True {
                      }
                    }
                  }
                }
                n483 = case shown="31" w500 {
                  tunnel: w508 -> [w552 w553 w554 w555 w556 w557 w558 w559 w560 w561 w562 w563 w564 w565 w566 w567 w568 w569 w570 w571 w572 w573 w574 w575 w576 w577 w578 w579 w580 w581 w582 w583]
                  frame 0, Default {
                    n484 = property on="light_1" class="Bool (严格)"("Colors [4]"=w552) -> ()  [unwired: 2 in, 2 out]
                  }
                  frame 1 {
                    n485 = property on="light_2" class="Bool (严格)"("Colors [4]"=w553) -> ()  [unwired: 2 in, 2 out]
                  }
                  frame 2 {
                    n486 = property on="light_3" class="Bool (严格)"("Colors [4]"=w554) -> ()  [unwired: 2 in, 2 out]
                  }
                  frame 3 {
                    n487 = property on="light_4" class="Bool (严格)"("Colors [4]"=w555) -> ()  [unwired: 2 in, 2 out]
                  }
                  frame 4 {
                    n488 = property on="light_5" class="Bool (严格)"("Colors [4]"=w556) -> ()  [unwired: 2 in, 2 out]
                  }
                  frame 5 {
                    n489 = property on="light_6" class="Bool (严格)"("Colors [4]"=w557) -> ()  [unwired: 2 in, 2 out]
                  }
                  frame 6 {
                    n490 = property on="light_7" class="Bool (严格)"("Colors [4]"=w558) -> ()  [unwired: 2 in, 2 out]
                  }
                  frame 7 {
                    n491 = property on="light_8" class="Bool (严格)"("Colors [4]"=w559) -> ()  [unwired: 2 in, 2 out]
                  }
                  frame 8 {
                    n492 = property on="light_9" class="Bool (严格)"("Colors [4]"=w560) -> ()  [unwired: 2 in, 2 out]
                  }
                  frame 9 {
                    n493 = property on="light_10" class="Bool (严格)"("Colors [4]"=w561) -> ()  [unwired: 2 in, 2 out]
                  }
                  frame 10 {
                    n494 = property on="light_11" class="Bool (严格)"("Colors [4]"=w562) -> ()  [unwired: 2 in, 2 out]
                  }
                  frame 11 {
                    n495 = property on="light_12" class="Bool (严格)"("Colors [4]"=w563) -> ()  [unwired: 2 in, 2 out]
                  }
                  frame 12 {
                    n496 = property on="light_13" class="Bool (严格)"("Colors [4]"=w564) -> ()  [unwired: 2 in, 2 out]
                  }
                  frame 13 {
                    n497 = property on="light_14" class="Bool (严格)"("Colors [4]"=w565) -> ()  [unwired: 2 in, 2 out]
                  }
                  frame 14 {
                    n498 = property on="light_15" class="Bool (严格)"("Colors [4]"=w566) -> ()  [unwired: 2 in, 2 out]
                  }
                  frame 15 {
                    n499 = property on="light_16" class="Bool (严格)"("Colors [4]"=w567) -> ()  [unwired: 2 in, 2 out]
                  }
                  frame 16 {
                    n500 = property on="light_17" class="Bool (严格)"("Colors [4]"=w568) -> ()  [unwired: 2 in, 2 out]
                  }
                  frame 17 {
                    n501 = property on="light_18" class="Bool (严格)"("Colors [4]"=w569) -> ()  [unwired: 2 in, 2 out]
                  }
                  frame 18 {
                    n502 = property on="light_19" class="Bool (严格)"("Colors [4]"=w570) -> ()  [unwired: 2 in, 2 out]
                  }
                  frame 19 {
                    n503 = property on="light_20" class="Bool (严格)"("Colors [4]"=w571) -> ()  [unwired: 2 in, 2 out]
                  }
                  frame 20 {
                    n504 = property on="light_21" class="Bool (严格)"("Colors [4]"=w572) -> ()  [unwired: 2 in, 2 out]
                  }
                  frame 21 {
                    n505 = property on="light_22" class="Bool (严格)"("Colors [4]"=w573) -> ()  [unwired: 2 in, 2 out]
                  }
                  frame 22 {
                    n506 = property on="light_23" class="Bool (严格)"("Colors [4]"=w574) -> ()  [unwired: 2 in, 2 out]
                  }
                  frame 23 {
                    n507 = property on="light_24" class="Bool (严格)"("Colors [4]"=w575) -> ()  [unwired: 2 in, 2 out]
                  }
                  frame 24 {
                    n508 = property on="light_25" class="Bool (严格)"("Colors [4]"=w576) -> ()  [unwired: 2 in, 2 out]
                  }
                  frame 25 {
                    n509 = property on="light_26" class="Bool (严格)"("Colors [4]"=w577) -> ()  [unwired: 2 in, 2 out]
                  }
                  frame 26 {
                    n510 = property on="light_27" class="Bool (严格)"("Colors [4]"=w578) -> ()  [unwired: 2 in, 2 out]
                  }
                  frame 27 {
                    n511 = property on="light_28" class="Bool (严格)"("Colors [4]"=w579) -> ()  [unwired: 2 in, 2 out]
                  }
                  frame 28 {
                    n512 = property on="light_29" class="Bool (严格)"("Colors [4]"=w580) -> ()  [unwired: 2 in, 2 out]
                  }
                  frame 29 {
                    n513 = property on="light_30" class="Bool (严格)"("Colors [4]"=w581) -> ()  [unwired: 2 in, 2 out]
                  }
                  frame 30 {
                    n514 = property on="light_31" class="Bool (严格)"("Colors [4]"=w582) -> ()  [unwired: 2 in, 2 out]
                  }
                  frame 31 {
                    n515 = property on="light_32" class="Bool (严格)"("Colors [4]"=w583) -> ()  [unwired: 2 in, 2 out]
                  }
                }
                n516 = case shown="31" w499 {
                  tunnel: w505 -> [w520 w521 w522 w523 w524 w525 w526 w527 w528 w529 w530 w531 w532 w533 w534 w535 w536 w537 w538 w539 w540 w541 w542 w543 w544 w545 w546 w547 w548 w549 w550 w551]
                  frame 0, Default {
                    n517 = property on="light_1" class="Bool (严格)"("Colors [4]"=w520) -> ()  [unwired: 2 in, 2 out]
                  }
                  frame 1 {
                    n518 = property on="light_2" class="Bool (严格)"("Colors [4]"=w521) -> ()  [unwired: 2 in, 2 out]
                  }
                  frame 2 {
                    n519 = property on="light_3" class="Bool (严格)"("Colors [4]"=w522) -> ()  [unwired: 2 in, 2 out]
                  }
                  frame 3 {
                    n520 = property on="light_4" class="Bool (严格)"("Colors [4]"=w523) -> ()  [unwired: 2 in, 2 out]
                  }
                  frame 4 {
                    n521 = property on="light_5" class="Bool (严格)"("Colors [4]"=w524) -> ()  [unwired: 2 in, 2 out]
                  }
                  frame 5 {
                    n522 = property on="light_6" class="Bool (严格)"("Colors [4]"=w525) -> ()  [unwired: 2 in, 2 out]
                  }
                  frame 6 {
                    n523 = property on="light_7" class="Bool (严格)"("Colors [4]"=w526) -> ()  [unwired: 2 in, 2 out]
                  }
                  frame 7 {
                    n524 = property on="light_8" class="Bool (严格)"("Colors [4]"=w527) -> ()  [unwired: 2 in, 2 out]
                  }
                  frame 8 {
                    n525 = property on="light_9" class="Bool (严格)"("Colors [4]"=w528) -> ()  [unwired: 2 in, 2 out]
                  }
                  frame 9 {
                    n526 = property on="light_10" class="Bool (严格)"("Colors [4]"=w529) -> ()  [unwired: 2 in, 2 out]
                  }
                  frame 10 {
                    n527 = property on="light_11" class="Bool (严格)"("Colors [4]"=w530) -> ()  [unwired: 2 in, 2 out]
                  }
                  frame 11 {
                    n528 = property on="light_12" class="Bool (严格)"("Colors [4]"=w531) -> ()  [unwired: 2 in, 2 out]
                  }
                  frame 12 {
                    n529 = property on="light_13" class="Bool (严格)"("Colors [4]"=w532) -> ()  [unwired: 2 in, 2 out]
                  }
                  frame 13 {
                    n530 = property on="light_14" class="Bool (严格)"("Colors [4]"=w533) -> ()  [unwired: 2 in, 2 out]
                  }
                  frame 14 {
                    n531 = property on="light_15" class="Bool (严格)"("Colors [4]"=w534) -> ()  [unwired: 2 in, 2 out]
                  }
                  frame 15 {
                    n532 = property on="light_16" class="Bool (严格)"("Colors [4]"=w535) -> ()  [unwired: 2 in, 2 out]
                  }
                  frame 16 {
                    n533 = property on="light_17" class="Bool (严格)"("Colors [4]"=w536) -> ()  [unwired: 2 in, 2 out]
                  }
                  frame 17 {
                    n534 = property on="light_18" class="Bool (严格)"("Colors [4]"=w537) -> ()  [unwired: 2 in, 2 out]
                  }
                  frame 18 {
                    n535 = property on="light_19" class="Bool (严格)"("Colors [4]"=w538) -> ()  [unwired: 2 in, 2 out]
                  }
                  frame 19 {
                    n536 = property on="light_20" class="Bool (严格)"("Colors [4]"=w539) -> ()  [unwired: 2 in, 2 out]
                  }
                  frame 20 {
                    n537 = property on="light_21" class="Bool (严格)"("Colors [4]"=w540) -> ()  [unwired: 2 in, 2 out]
                  }
                  frame 21 {
                    n538 = property on="light_22" class="Bool (严格)"("Colors [4]"=w541) -> ()  [unwired: 2 in, 2 out]
                  }
                  frame 22 {
                    n539 = property on="light_23" class="Bool (严格)"("Colors [4]"=w542) -> ()  [unwired: 2 in, 2 out]
                  }
                  frame 23 {
                    n540 = property on="light_24" class="Bool (严格)"("Colors [4]"=w543) -> ()  [unwired: 2 in, 2 out]
                  }
                  frame 24 {
                    n541 = property on="light_25" class="Bool (严格)"("Colors [4]"=w544) -> ()  [unwired: 2 in, 2 out]
                  }
                  frame 25 {
                    n542 = property on="light_26" class="Bool (严格)"("Colors [4]"=w545) -> ()  [unwired: 2 in, 2 out]
                  }
                  frame 26 {
                    n543 = property on="light_27" class="Bool (严格)"("Colors [4]"=w546) -> ()  [unwired: 2 in, 2 out]
                  }
                  frame 27 {
                    n544 = property on="light_28" class="Bool (严格)"("Colors [4]"=w547) -> ()  [unwired: 2 in, 2 out]
                  }
                  frame 28 {
                    n545 = property on="light_29" class="Bool (严格)"("Colors [4]"=w548) -> ()  [unwired: 2 in, 2 out]
                  }
                  frame 29 {
                    n546 = property on="light_30" class="Bool (严格)"("Colors [4]"=w549) -> ()  [unwired: 2 in, 2 out]
                  }
                  frame 30 {
                    n547 = property on="light_31" class="Bool (严格)"("Colors [4]"=w550) -> ()  [unwired: 2 in, 2 out]
                  }
                  frame 31 {
                    n548 = property on="light_32" class="Bool (严格)"("Colors [4]"=w551) -> ()  [unwired: 2 in, 2 out]
                  }
                }
              }
              frame #2 {
                n549 = local read "第几组数据"() -> (w587:i32)
                n550 = Add(x=w587, y=16) -> (x+y=w589:i32)
                n551 = local read "第几个数据"() -> (w591:i32)
                n552 = local read "合格？"() -> (w592:bool[][])
                n553 = local read "数组_选择"() -> (w590:bool[])
                n554 = Index Array(array=w592, index (row) #1=w587, index (col) #1=w591, index (row) #2=w589, index (col) #2=w591) -> (element #1=w588:bool, element #2=w584:bool)
                n555 = Index Array(array=w590, index #1=w587, index #2=w589) -> (element #1=w586:bool, element #2=w585:bool)
                n556 = case shown="真" w586 {
                  tunnel: w591 -> [_ w603]
                  tunnel: w588 -> [_ w602]
                  tunnel: w587 -> [_ w601]
                  frame False {
                  }
                  frame True {
                    n557 = call "误差表格颜色.vi"("合格？"=w602, "第几组"=w601) -> ("颜色"=w600:u32)  [unwired: 9 in]
                    n558 = Bundle("第几组数据"=w601, "第几个数据"=w603) -> (w605:cluster{"第几组数据":i32, "第几个数据":i32})  [unwired: 1 in]
                    n559 = property on="Analog_WC" class="Tbl (严格)"("Active Cell"=w605) -> (error out=w604:errorcluster)  [unwired: 2 in, 1 out]
                    n560 = property on="Analog_WC" class="Tbl (严格)"(error in=w604, "Cell BG Color"=w600) -> ()  [unwired: 1 in, 2 out]
                  }
                }
                n561 = case shown="真" w585 {
                  tunnel: w591 -> [_ w597]
                  tunnel: w589 -> [_ w596]
                  tunnel: w584 -> [_ w594]
                  frame False {
                  }
                  frame True {
                    n562 = Bundle(w596, "第几个数据"=w597) -> (w598:cluster{i32, "第几个数据":i32})  [unwired: 1 in]
                    n563 = call "误差表格颜色.vi"("合格？"=w594, "第几组"=w596) -> ("颜色"=w595:u32)  [unwired: 9 in]
                    n564 = property on="Analog_WC" class="Tbl (严格)"("Active Cell"=w598) -> (error out=w599:errorcluster)  [unwired: 2 in, 1 out]
                    n565 = property on="Analog_WC" class="Tbl (严格)"(error in=w599, "Cell BG Color"=w595) -> ()  [unwired: 1 in, 2 out]
                  }
                }
              }
              frame #3 {
                n566 = flat-sequence {
                  frame #0 {
                    n567 = Wait Until Next ms Multiple(millisecond multiple=u32 100) -> ()  [unwired: 1 out]
                  }
                  frame #1 {
                    n568 = local write "同步_1"(0 ("同步_1")) -> ()
                  }
                }
              }
            }
          }
        }
        n569 = case shown="真" w439 {
          frame False {
          }
          frame True {
            # "第几个"
            # "第几组"
            n570 = local read "第几个数据"() -> (w450:i32)
            n571 = local read "第几组数据"() -> (w452:i32)
            n572 = Increment(x=w452) -> (x+1=w453:i32)
            n573 = Increment(x=w450) -> (x+1=w451:i32)
            n574 = Format Into String(format string="第%d组%d个数据反馈失败（UDP）" ("Message"), w453, w451) -> (resulting string=w454:string)  [unwired: 2 in, 1 out]
            n575 = call "显示对话框信息2"("Message"=w454) -> ()  [unwired: 9 in, 2 out]
            n576 = local write "同步_1"(0 ("同步_1")) -> ()
          }
        }
      }
    }
    n577 = local read "退出？"() -> (w425:bool)
  }
  n578 = Release Notifier(notifier=w2, error in (no error)=w1) -> ()  [unwired: 1 in, 3 out]
